vi "AI Readback All.vi"(7 "Box ID":u8=1, 8 "error in (no error)":errorcluster, 11 "CAN in":refnum<class "XNET_BS120x.lvclass">) -> (0 "error out":errorcluster, 2 "Voltage":dbl[](array[numeric]), 3 "CAN out":refnum<class "XNET_BS120x.lvclass">)   [LabVIEW 2021, in "BS120x Driver.lvlib" / "XNET_BS120x.lvclass"]
uses:
  XNET_BS120x.lvclass
  BS120x.lvclass
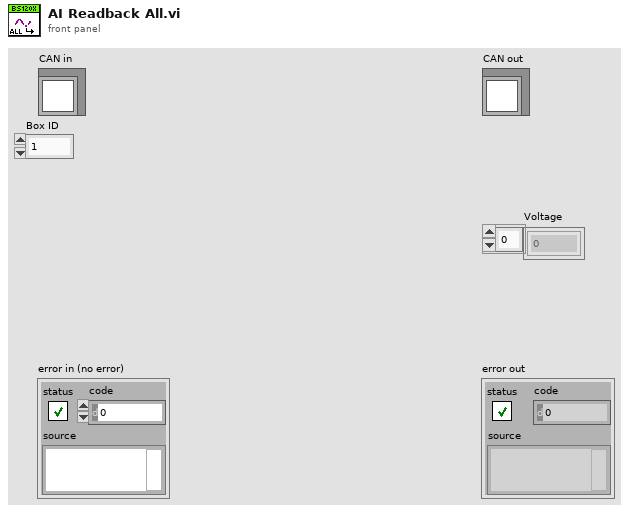
[diagram p1: front panel]
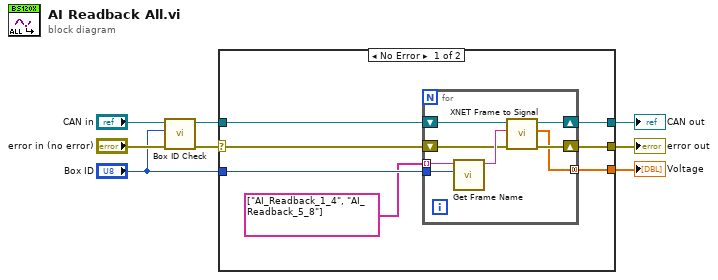
[diagram p0: block diagram]
diagram:
  n1 = call "Box ID Check.vi"("error in (no error)"="error in (no error)", "Box ID"="Box ID", "CAN in"="CAN in") -> ("error out"=w3:errorcluster, "CAN out"=w5:refnum<class "XNET_BS120x.lvclass">)  [unwired: 7 in]
  n2 = case shown="No Error" w3 {
    selector: w3 -> [w13 w25]
    tunnel: w5 -> [w15 w24]
    tunnel: [w11 w24] -> w8
    tunnel: [w10 w25] -> w7
    tunnel: "Box ID" -> [w14 _]
    tunnel: [w9 _] -> w1
    frame No Error {
      n3 = for {
        tunnel: w14 -> [w21]
        tunnel: string[] ["AI_Readback_1_4", "AI_Readback_5_8"] -> [w19] mode=indexing
        shift-right: [w18] -> w11
        shift-left: w15 -> [w23]
        shift-right: [w17] -> w10
        shift-left: w13 -> [w20]
        tunnel: [w16] -> w9 mode=concatenating
        n4 = call "Get Frame Name.vi"("Box ID"=w21, "Frame Name"=w19) -> ("Frame Name out"=w22:string)  [unwired: 9 in]
        n5 = call "XNET Frame to Signal.vi"("error in (no error)"=w20, "Frame"=w22, "CAN in"=w23) -> ("error out"=w17:errorcluster, "signal data"=w16:dbl[], "CAN out"=w18:refnum<class "XNET_BS120x.lvclass">)  [unwired: 6 in]
      }
    }
    frame Error {
    }
  }
  "error out" <- w7
  "CAN out" <- w8
  "Voltage" <- w1
